vi "Global-Var-OperService.vi"() -> ()   [LabVIEW 2021]
panel:
  out "delete_all_external_alarms_G":bool
  out "service_WorkFinished_G":bool
  out "service_WorkStarted_G":bool
  out "service_Received_G":bool
  out "service_Sent_G":bool
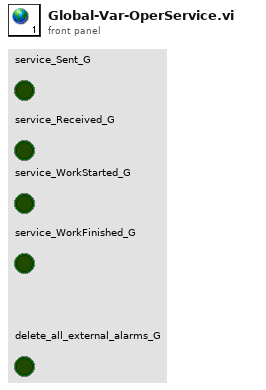
[diagram p1: front panel]
diagram:
